vi "dialog save before deploy.vi"(8 "error in":errorcluster, 9 "View":refnum<vi>, 11 "state in":T1) -> (0 "error out":errorcluster, 1 "Continue?":bool, 3 "state out":T1)   [LabVIEW 2013, in "Standard Editor.lvlib"]
uses:
  Standard Editor.lvlib
  Controls/StateCluster.ctl
  Configuration Editor/Classes/SystemConfigRepo/SystemConfigRepo.lvclass
  Configuration Editor/Classes/Systems/Systems.lvclass
  <vilib>/NI/Configuration Framework/Node/StandardEvents.ctl
  <vilib>/NI/Configuration Framework/Node/UserEventRef.ctl
  <vilib>/NI/Configuration Framework/Controls/EventCluster.ctl
  <vilib>/NI/Configuration Framework/Node/NodeChangeEvent.ctl
  <vilib>/NI/Configuration Framework/Node/NodeRef.ctl
  <vilib>/NI/Configuration Framework/Node/NISE_CEF_Node.lvclass
  <vilib>/NI/Configuration Framework/Node/CacheState.ctl
  <vilib>/NI/Configuration Framework/Node/RefreshUIEvent.ctl
  <vilib>/NI/Configuration Framework/Node/StopEvent.ctl
  <vilib>/NI/Configuration Framework/glyph manager/glyph manager.ctl
  <vilib>/picture/picture.llb/imagedata.ctl
  <vilib>/NI/AMC/Message Queue.ctl
  <vilib>/NI/AMC/Message.ctl
  <vilib>/NI/Tools/Keyed Array/KeyedArray.ctl
  <vilib>/NI/Configuration Framework/NISE_CEF_TreeControl.lvlib
  <vilib>/NI/Configuration Framework/glyph manager/glyph manager.lvlib
  <vilib>/NI/Tools/Keyed Array/Tools_KeyedArray.lvlib
  <vilib>/NI/AMC/AMC.lvlib
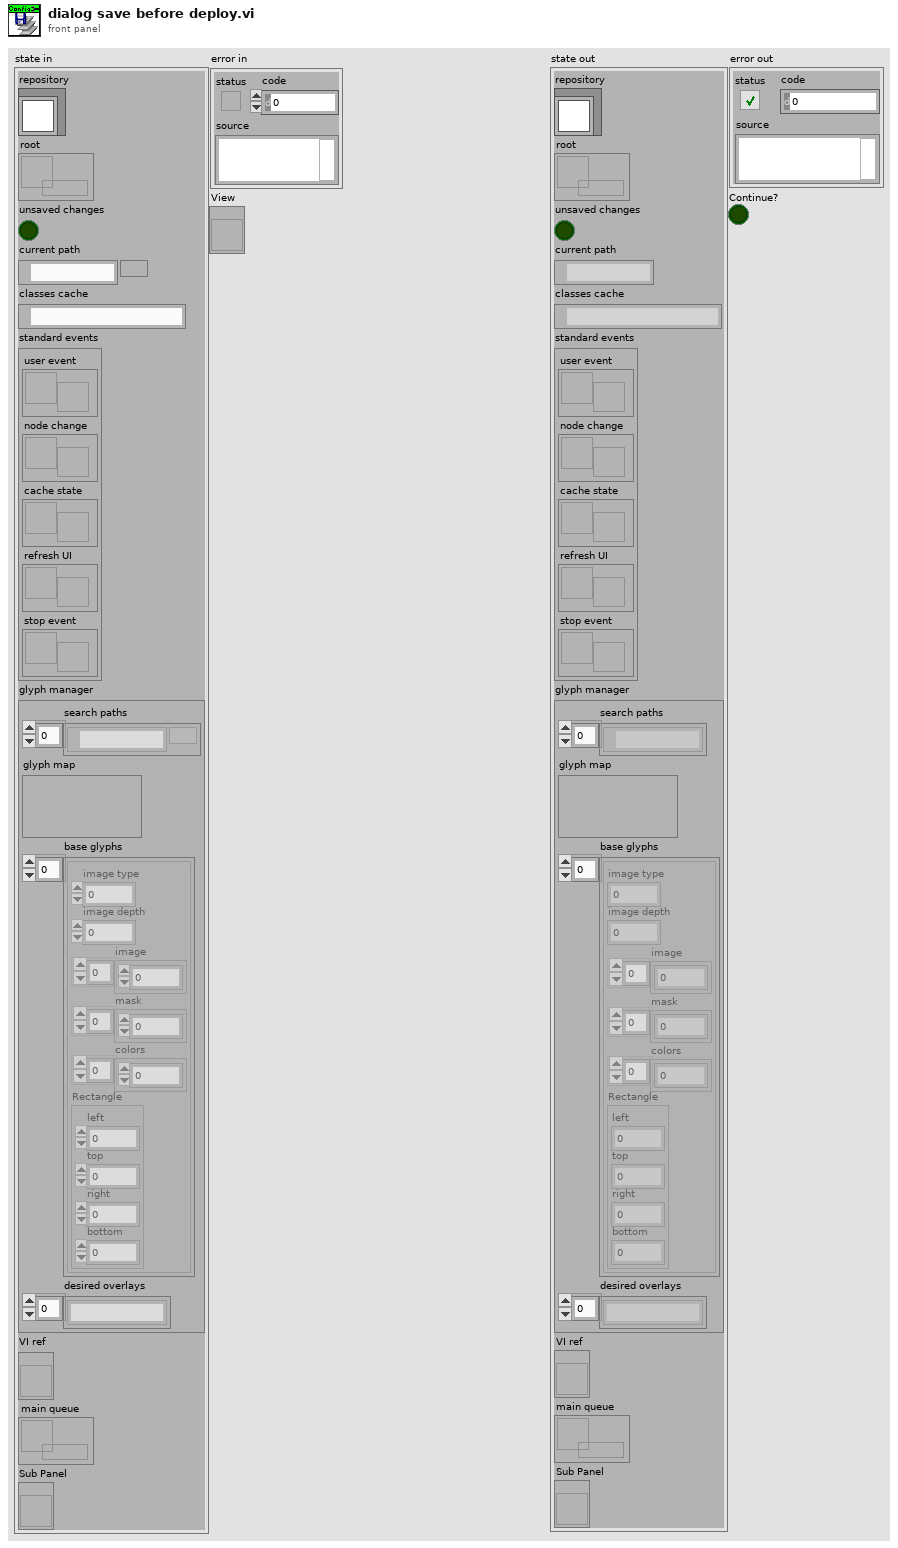
[diagram p1: front panel]
types:
  T1 = typedef "Standard Editor.lvlib/StateCluster.ctl" = cluster{"repository":refnum<class "SystemConfigRepo.lvclass">, "root":refnum<data-value>, "unsaved changes":bool, "current path":path, "classes cache":path, "standard events":T2, "glyph manager":T8, "VI ref":refnum<vi>, "main queue":T10, "Sub Panel":refnum<vi>}
  T2 = typedef "NISE_CEF_Node.lvclass/StandardEvents.ctl" = cluster{"user event":T3, "node change":T4, "cache state":T5, "refresh UI":T6, "stop event":T7}
  T3 = typedef "NISE_CEF_Node.lvclass/UserEventRef.ctl" = refnum<user-event>
  T4 = typedef "NISE_CEF_Node.lvclass/NodeChangeEvent.ctl" = refnum<user-event>
  T5 = typedef "NISE_CEF_Node.lvclass/CacheState.ctl" = refnum<user-event>
  T6 = typedef "NISE_CEF_Node.lvclass/RefreshUIEvent.ctl" = refnum<user-event>
  T7 = typedef "NISE_CEF_Node.lvclass/StopEvent.ctl" = refnum<user-event>
  T8 = typedef "glyph manager.lvlib/glyph manager.ctl" = cluster{"search paths":path[], "glyph map":variant, "base glyphs":T9[], "desired overlays":string[]}
  T9 = typedef "imagedata.ctl" = cluster{"image type":i32, "image depth":i32, "image":u8[], "mask":u8[], "colors":u32[], "Rectangle":cluster{"left":i16, "top":i16, "right":i16, "bottom":i16}}
  T10 = typedef "AMC.lvlib/Message Queue.ctl" = refnum<queue>
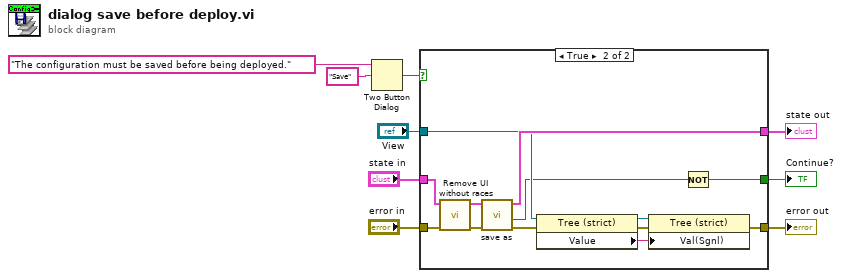
[diagram p0: block diagram]
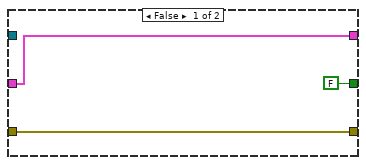
[diagram p2: hidden frame]
diagram:
  n1 = Two Button Dialog(message="The configuration must be saved before being deployed.", 2:"Save" ("T button name (\"OK\")")) -> (T button?=w7:bool)  [unwired: 1 in]
  n2 = case shown="True" w7 {
    tunnel: "state in" -> [w12 w23]
    tunnel: [w12 w22] -> w5
    tunnel: "error in" -> [w11 w21]
    tunnel: [w11 w16] -> w3
    tunnel: "View" -> [_ w17]
    tunnel: [FALSE w14] -> w1
    frame False {
    }
    frame True {
      n3 = call "Remove UI without races.vi"("error in"=w21, "state in"=w23) -> ("error out"=w24:errorcluster, "state out"=w25:T1)  [unwired: 8 in]
      n4 = call "save as.vi"("error in"=w24, "state in"=w25) -> ("error out"=w18:errorcluster, "canceled?"=w15:bool, "state out"=w22:T1)  [unwired: 7 in]
      n5 = property class="Tree (strict)"(reference=w17, error in=w18) -> (reference out=w13:refnum<vi>, error out=w20:errorcluster, "Value"=w19:string)
      n6 = property class="Tree (strict)"(reference=w13, error in=w20, "Val(Sgnl)"=w19) -> (error out=w16:errorcluster)  [unwired: 1 out]
      n7 = Not(x=w15) -> (.not. x?=w14:bool)
    }
  }
  "state out" <- w5
  "error out" <- w3
  "Continue?" <- w1
